vi "Check Comment Line.vi"(1 "String":string) -> (0 "Starts with #?":bool)   [LabVIEW 2013]
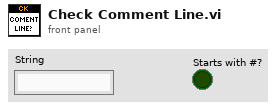
[diagram p1: front panel]
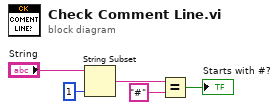
[diagram p0: block diagram]
diagram:
  n1 = String Subset(string="String", length (rest)=1 ("length (rest)")) -> (substring=w3:string)  [unwired: 1 in]
  n2 = Equal?(x=w3, y="#") -> (x = y?=→"Starts with #?":bool)
